vi "FeatureA.vi"(8 "error in (no error)":errorcluster, 11 "SimpleDevice in":refnum<class "SimpleDevice.lvclass">) -> (0 "error out":errorcluster, 3 "SimpleDevice out":refnum<class "SimpleDevice.lvclass">)   [LabVIEW 2021, in "SimpleDevice.lvlib" / "SimpleDevice.lvclass"]
uses:
  SimpleDevice.lvclass
  SimpleDevice.lvclass/SimpleDevice.ctl
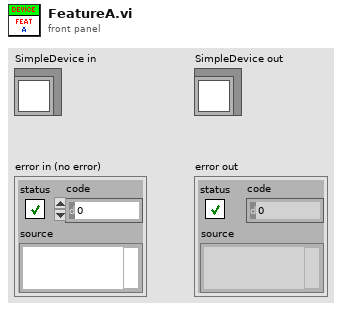
[diagram p1: front panel]
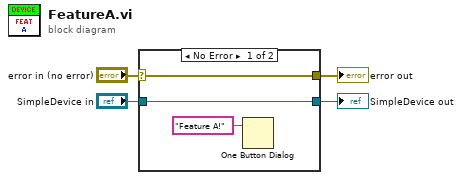
[diagram p0: block diagram]
diagram:
  n1 = case shown="No Error" "error in (no error)" {
    selector: "error in (no error)" -> [w6 w9]
    tunnel: [w6 w9] -> w3
    tunnel: [w7 w8] -> w1
    tunnel: "SimpleDevice in" -> [w7 w8]
    frame No Error {
      n2 = One Button Dialog(message="Feature A!") -> ()  [unwired: 1 in, 1 out]
    }
    frame Error {
    }
  }
  "error out" <- w3
  "SimpleDevice out" <- w1
